vi "magnetoresistance.vi"() -> ()   [LabVIEW 2017]
doc: "Use this template to build a simple state machine design pattern. Each state executes code and determines which state to transition to."
uses:
  controls/State.ctl
  controls/Instruments.ctl
  controls/State_of_loop.ctl
  controls/Data.ctl
  <vilib>/Utility/error.llb/DialogType.ctl
  <vilib>/DAQmx/write.llb/DAQmx Write (Analog DBL 1Chan 1Samp).vi
  <vilib>/DAQmx/create/channels.llb/DAQmx Create Channel (AO-Voltage-Basic).vi
  <vilib>/DAQmx/create/channels.llb/DAQmx Create Channel (AI-Voltage-Basic).vi
  <vilib>/DAQmx/configure/timing.llb/DAQmx Timing (Sample Clock).vi
  <vilib>/DAQmx/configure/trigger.llb/DAQmx Start Trigger (None).vi
  <vilib>/DAQmx/miscellaneous.llb/DAQmx Fill In Error Info.vi
panel:
  in  "Number of loops":i32=1 caption="Stop H Field (Oe)" min=0
  in  "Time to wait, ms":i32=100 caption="Stop H Field (Oe)" min=0
  in  "Clear button":bool
  in  "Data Type":T1(ring)=enum."Resistance, Ohm"
  out "Ush.Min":dbl=-0.5
  out "Ush.Max":dbl=0.5
  out "U.Min":dbl=-0.5
  out "U.Max":dbl=0.5
  in  "Load resistance, Ohm":dbl=2351.0 min=0.0
  in  "Switch port":refnum<visa-resource-name>="COM6"
  in  "AKIP":refnum<visa-resource-name>="AKIP"
  in  "DAQ channel Voltage Output":tag="DAQ6363/ao0"
  in  "DAQ channel Voltage U":tag="DAQ6363/ai5"
  in  "DAQ channel Voltage Ush":tag="DAQ6363/ai4"
  in  "Resolution, Oe/point":dbl=50.0 caption="Stop H Field (Oe)" min=0.0 format="%#_6f"
  out "DC power electromagnet":cluster{"Voltage":dbl, "Current":dbl}={"Voltage"=0.005, "Current"=0.05} {"Voltage" format="%.2f"; "Current" format="%.2f"}
  out "Error Out":errorcluster={"status"=FALSE, "code"=1073676293, "source"="VISA Read in AKIP_read.vi->AKIP_error_check.vi->AKIP_reset_errors.vi->magnetoresistance.vi"}
  in  "Error In (no error)":errorcluster
  in  "Voltage Output, V":dbl=0.5 min=0.0 max=5.0
  in  "H Field Max, Oe":dbl=1200.0 caption="Stop H Field (Oe)" min=0.0 max=6000.0 format="%#_6f"
  in  "H Field Min, Oe":dbl=-1200.0 min=-6000.0 max=0.0 format="%#_6f"
  out "Status":string="Shutting down..."
  in  "Exit Button":bool
  in  "Save Button":bool
  out "Cursor":cluster{"x":dbl, "y":dbl} {"x" format="%.2f"; "y" format="%.5f"}
  out "SpectrumGraph":cluster{"Old Field":dbl[], "Old Signal":dbl[]}[](graph)
  in  "Start Button":bool
  in  "Stop Button":bool
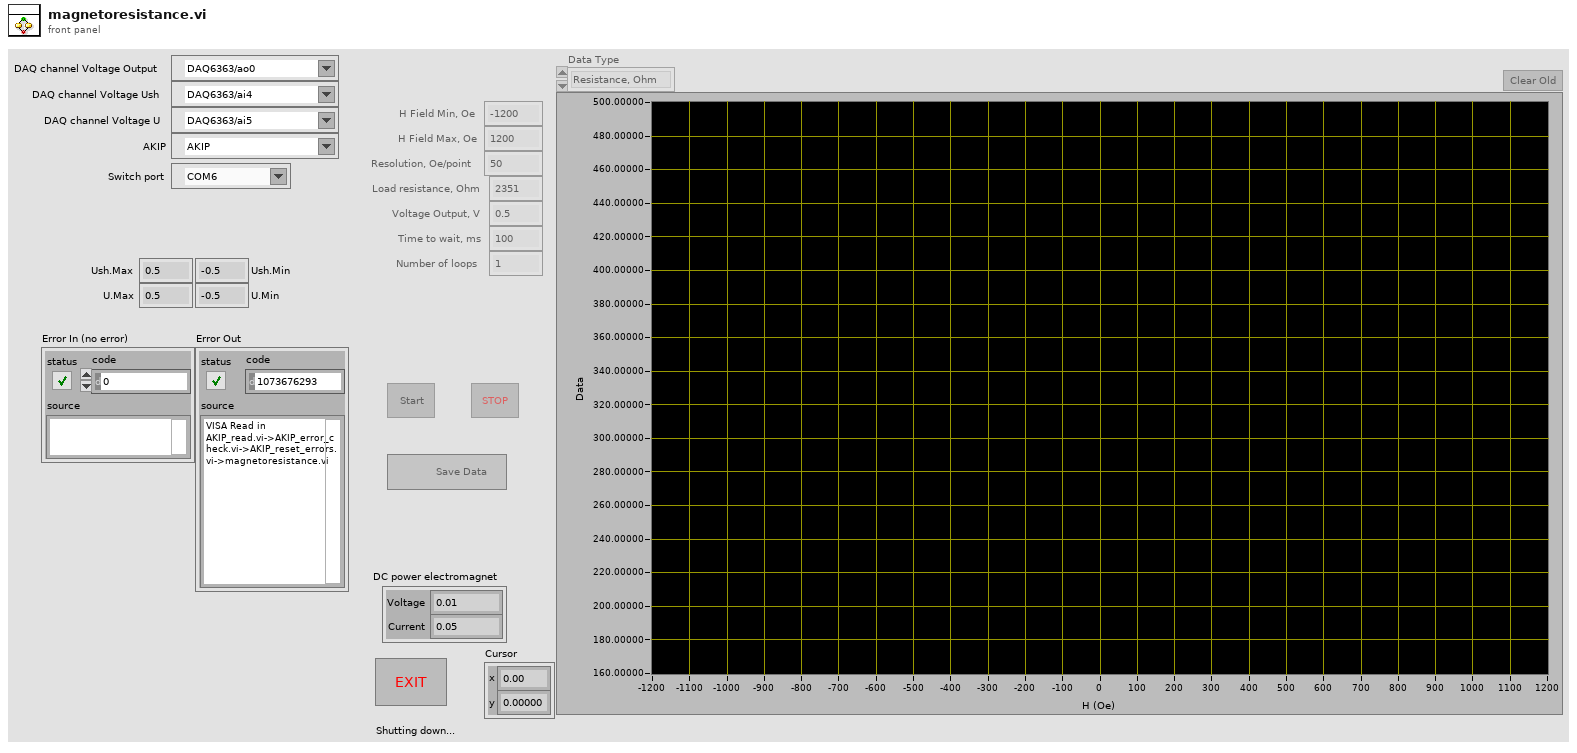
[diagram p1: front panel]
types:
  T1 = enum16{"Voltage Ush, V", "Voltage U, V", "Sum Voltage, V", "Current, mA", "Resistance, Ohm"}
  T2 = typedef "Data.ctl" = cluster{"Field":dbl[], "Voltage Ush":dbl[], "Voltage U":dbl[], "Sum Voltage":dbl[], "Current":dbl[], "Resistance":dbl[], "Old Field":dbl[], "Old Voltage Ush":dbl[], "Old Voltage U":dbl[], "Old Sum Voltage":dbl[], "Old Current":dbl[], "Old Resistance":dbl[]}
  T3 = typedef "State_of_loop.ctl" = enum16{"from zero to max", "from max to zero", "from zero to min", "from min to zero"}
  T4 = typedef "Instruments.ctl" = cluster{"DAQ AO task":refnum<k21>, "DAQ AI task":refnum<k21>, "DAQ channel Voltage Output":tag, "DAQ channel Voltage U":tag, "DAQ channel Voltage Ush":tag, "AKIP":refnum<visa-resource-name>, "Switch port":refnum<visa-resource-name>}
  T5 = typedef "State.ctl" = enum16{"Init", "Idle", "Starting meas", "Running", "Stopping meas", "Shutdown"}
  T6 = cluster{"Old Field":dbl[], "Old Resistance":dbl[]}[]
  T7 = cluster{"Voltage Ush":dbl, "Voltage U":dbl, "Sum Voltage":dbl, "Current":dbl, "Resistance":dbl}
  T8 = typedef "DialogType.ctl" = u16
  T9 = typedef "LVPoint32TypeDef.ctl" = cluster{"Horizontal":i32, "Vertical":i32}
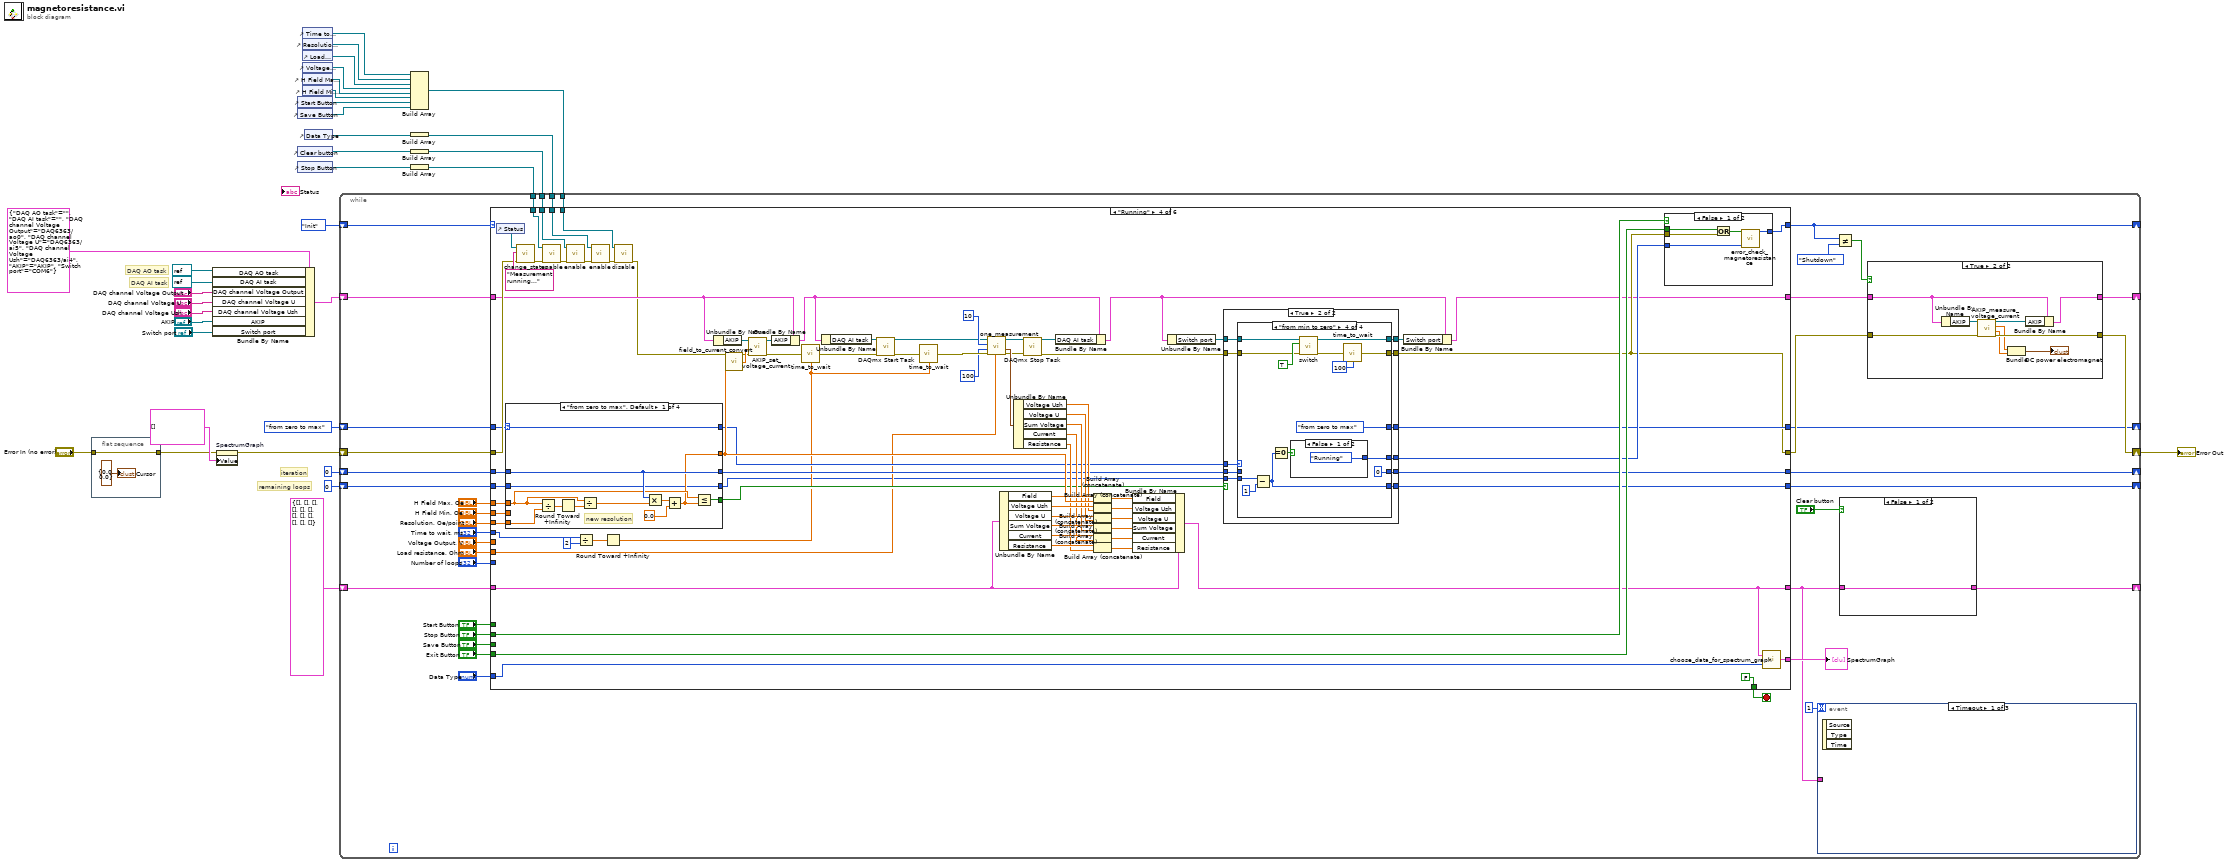
[diagram p0: block diagram]
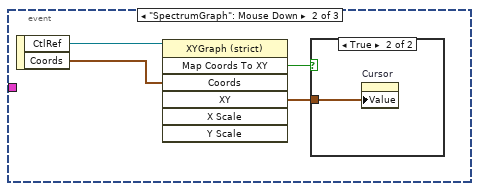
[diagram p3: hidden frame]
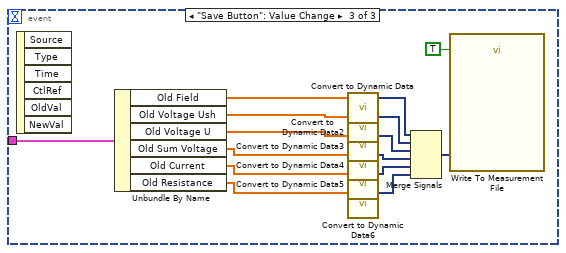
[diagram p5: hidden frame]
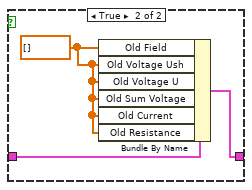
[diagram p6: hidden frame]
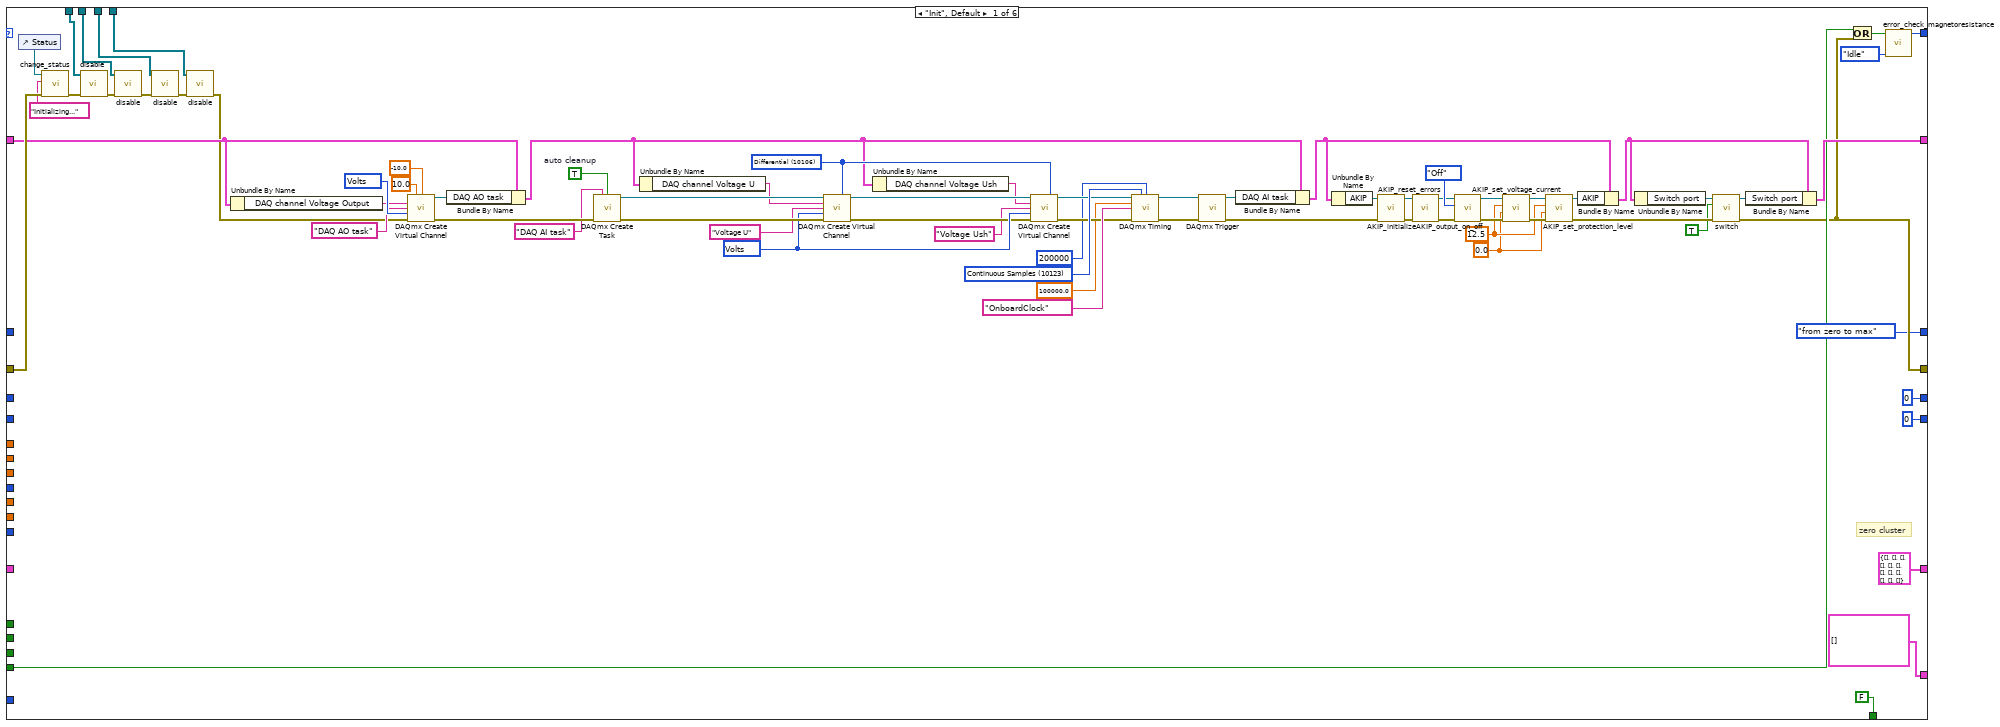
[diagram p7: hidden frame]
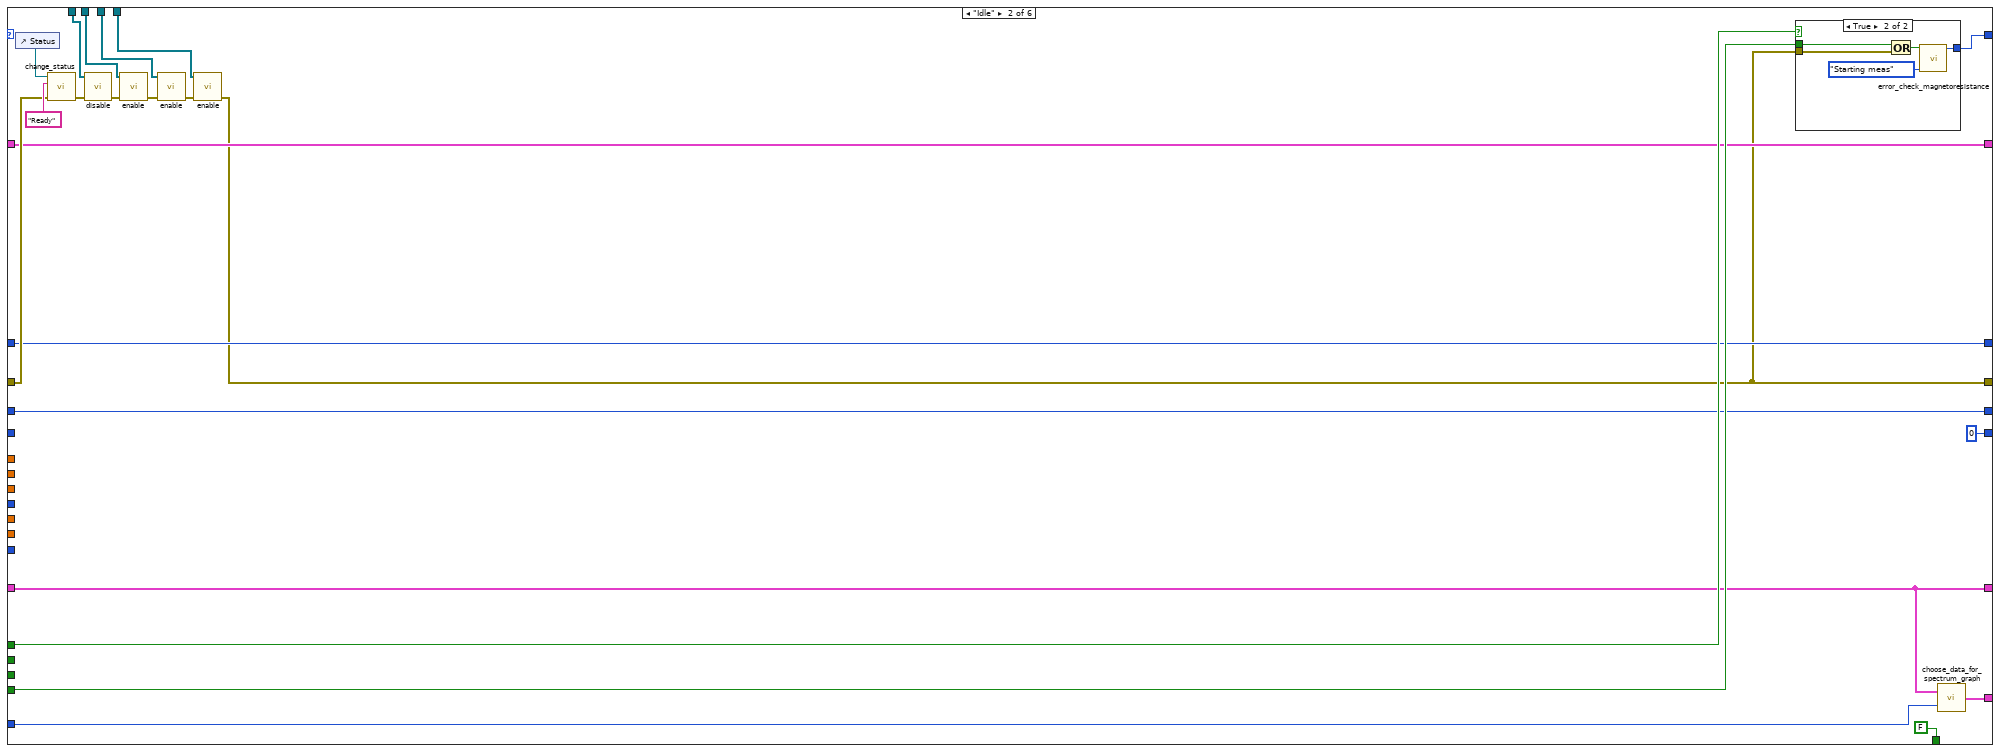
[diagram p8: hidden frame]
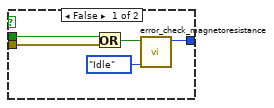
[diagram p9: hidden frame]
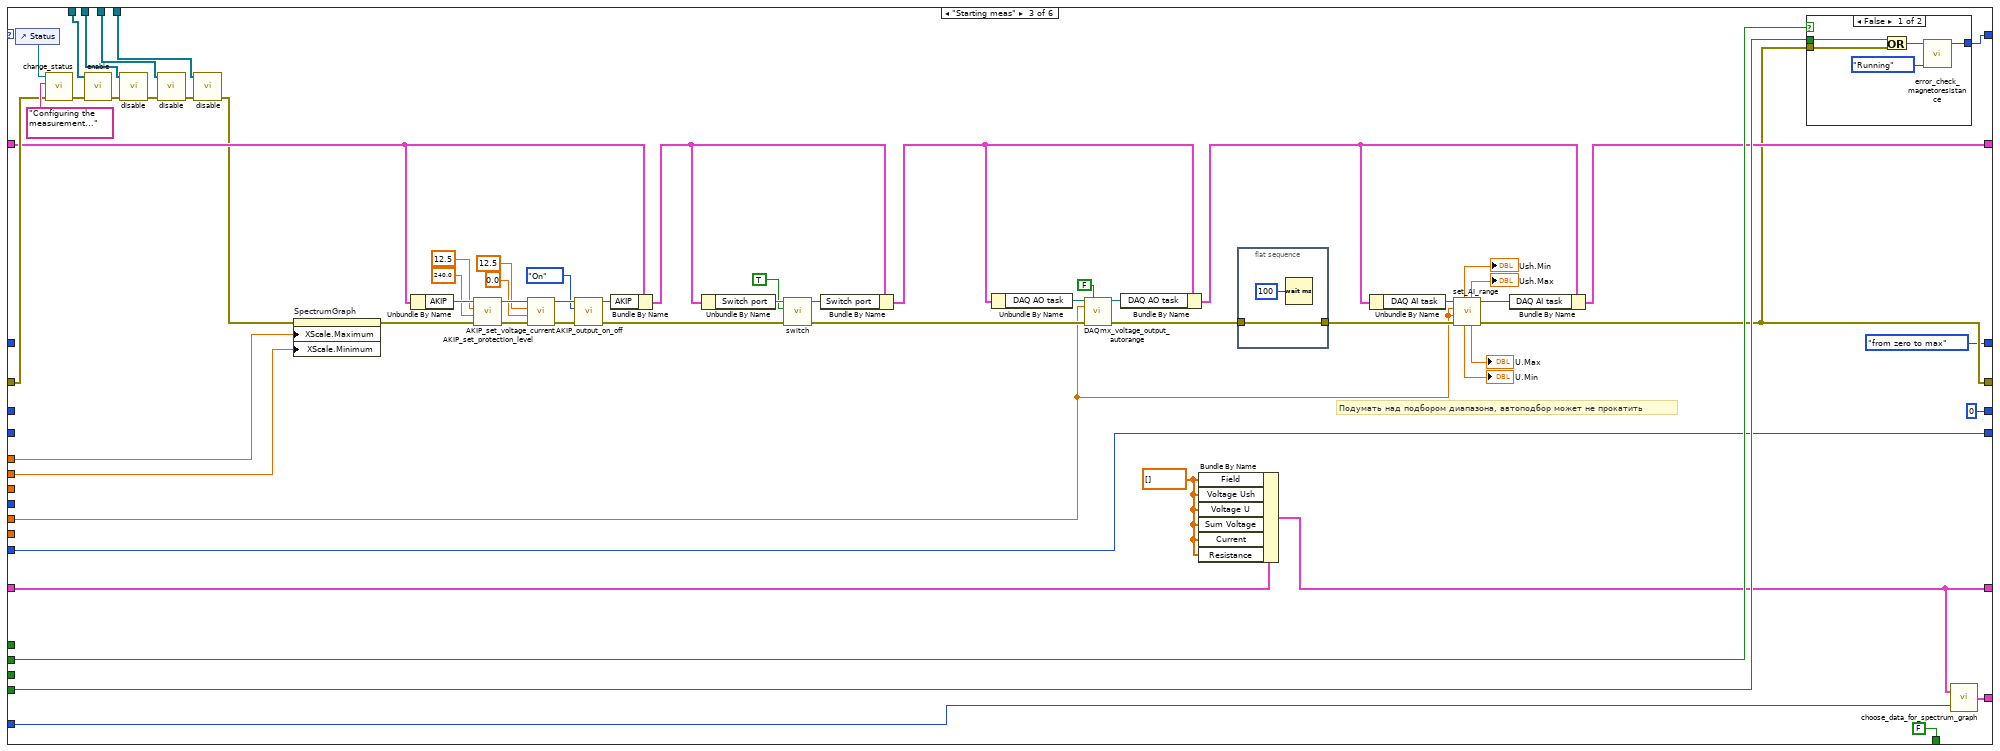
[diagram p10: hidden frame]
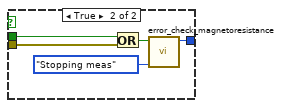
[diagram p11: hidden frame]
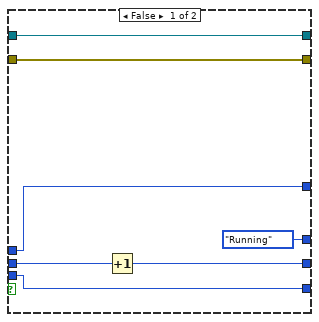
[diagram p12: hidden frame]
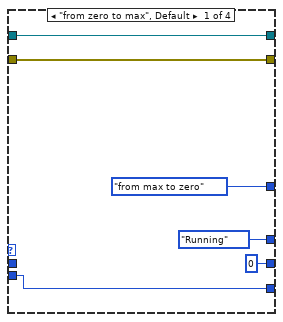
[diagram p13: hidden frame]
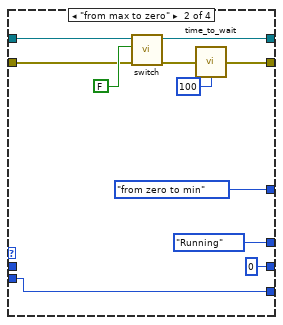
[diagram p14: hidden frame]
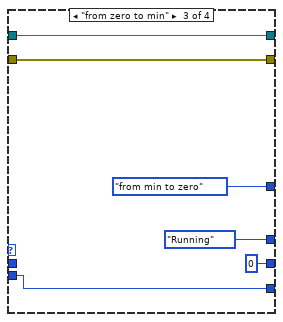
[diagram p15: hidden frame]
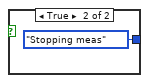
[diagram p16: hidden frame]
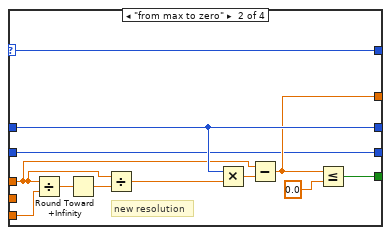
[diagram p17: hidden frame]
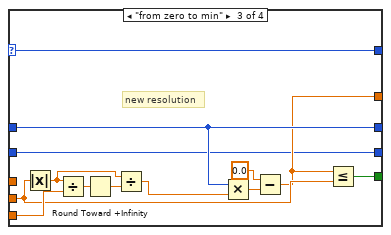
[diagram p18: hidden frame]
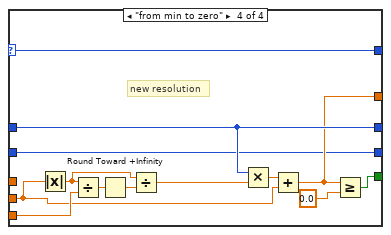
[diagram p19: hidden frame]
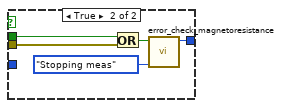
[diagram p20: hidden frame]
diagram:
  # "iteration"
  # "remaining loops"
  # "DAQ AI task"
  # "DAQ AO task"
  n1 = flat-sequence {
    tunnel: "Error In (no error)" -> [w36]
    tunnel: [w36] -> w23
    frame #0 {
      "Cursor" <- cluster{"x":dbl, "y":dbl} {"x"=0.0, "y"=0.0} ("Cursor")
    }
  }
  n2 = Bundle By Name(cluster=T4 {"DAQ AO task"="", "DAQ AI task"="", "DAQ channel Voltage Output"="DAQ6363/ao0", "DAQ channel Voltage U"="DAQ6363/ai5", "DAQ channel Voltage Ush"="DAQ6363/ai4", "AKIP"="AKIP", "Switch port"="COM6"} ("Cluster"), "DAQ AO task"=refnum<k21> refnum ("task in"), "DAQ AI task"=refnum<k21> refnum ("task out"), "DAQ channel Voltage Output"="DAQ channel Voltage Output", "DAQ channel Voltage U"="DAQ channel Voltage U", "DAQ channel Voltage Ush"="DAQ channel Voltage Ush", "AKIP"="AKIP", "Switch port"="Switch port") -> (w15:T4)
  n3 = property on="SpectrumGraph" class="XYGraph (strict)"(error in=w23, "Value"=cluster{"Old Field":dbl[], "Old Signal":dbl[]}[] [] ("SpectrumGraph")) -> (error out=w27:errorcluster)  [unwired: 1 in, 1 out]
  n4 = control-ref of="Start Button"() -> (w32:refnum<vi>)
  n5 = control-ref of="Save Button"() -> (w31:refnum<vi>)
  n6 = control-ref of="Clear button"() -> (w9:refnum<vi>)
  n7 = control-ref of="Stop Button"() -> (w30:refnum<vi>)
  n8 = control-ref of="Time to wait, ms"() -> (w2:refnum<vi>)
  n9 = control-ref of="Resolution, Oe/point"() -> (w3:refnum<vi>)
  n10 = control-ref of="Load resistance, Ohm"() -> (w4:refnum<vi>)
  n11 = control-ref of="Voltage Output, V"() -> (w5:refnum<vi>)
  n12 = control-ref of="H Field Max, Oe"() -> (w34:refnum<vi>)
  n13 = control-ref of="H Field Min, Oe"() -> (w33:refnum<vi>)
  n14 = control-ref of="Data Type"() -> (w8:refnum<vi>)
  n15 = Build Array(w2, w3, w4, w5, w34, w33, w32, w31) -> (w28:refnum<vi>[])
  n16 = Build Array(w8) -> (w7:refnum<vi>[])
  n17 = Build Array(w9) -> (w6:refnum<vi>[])
  n18 = Build Array(w30) -> (w29:refnum<vi>[])
  n19 = while {
    tunnel: w29 -> [w75]
    tunnel: w28 -> [w74]
    shift-right: [w43] -> _
    shift-left: State."Init" ("States") -> [w68]
    shift-right: [w62] -> w14
    shift-left: w27 -> [w73]
    shift-right: [w64] -> _
    shift-left: w15 -> [w66]
    shift-right: [w55] -> _
    shift-left: State_of_loop."from zero to max" -> [w56]
    shift-right: [w53] -> _
    shift-left: 0 -> [w54]
    shift-right: [w48] -> _
    shift-left: T2 {"Field"=[], "Voltage Ush"=[], "Voltage U"=[], "Sum Voltage"=[], "Current"=[], "Resistance"=[], "Old Field"=[], "Old Voltage Ush"=[], "Old Voltage U"=[], "Old Sum Voltage"=[], "Old Current"=[], "Old Resistance"=[]} ("SpectrumGraph") -> [w52]
    tunnel: w6 -> [w45]
    tunnel: w7 -> [w44]
    shift-right: [w37] -> _
    shift-left: 0 -> [w38]
    stop <- w67 stop-if-true
    n20 = case shown="\"Running\"" w68 {
      tunnel: w75 -> [w115 w189 w228 w307 w493 w548]
      tunnel: w74 -> [w112 w186 w225 w304 w490 w545]
      tunnel: w73 -> [w183 w206 w277 w368 w541 w595]
      tunnel: "Start Button" -> [_ w204 _ _ _ _]
      tunnel: "Stop Button" -> [_ _ w252 w366 _ _]
      tunnel: "Save Button" -> [_ _ _ _ _ _]
      tunnel: "Exit Button" -> [w122 w203 w251 w365 w509 _]
      tunnel: [w174 w202 w253 w367 w511 State."Shutdown" ("States out")] -> w43
      tunnel: [FALSE FALSE FALSE FALSE FALSE TRUE] -> w67
      tunnel: w66 -> [w165 w200 w242 w356 w523 w578]
      tunnel: [w123 w200 w249 w319 w514 w570] -> w65
      tunnel: [w121 w190 w248 w323 w510 w577] -> w63
      tunnel: "Load resistance, Ohm" -> [_ _ _ w294 _ _]
      tunnel: "H Field Max, Oe" -> [_ _ w222 w361 _ _]
      tunnel: "H Field Min, Oe" -> [_ _ w221 w360 _ _]
      tunnel: "Voltage Output, V" -> [_ _ w219 _ _ _]
      tunnel: "Resolution, Oe/point" -> [_ _ _ w359 _ _]
      tunnel: w56 -> [_ w199 _ w364 _ _]
      tunnel: [State_of_loop."from zero to max" w199 State_of_loop."from zero to max" w324 State_of_loop."from zero to max" State_of_loop."from zero to max"] -> w55
      tunnel: w54 -> [_ w195 _ w363 _ _]
      tunnel: [0 w195 0 w328 0 0] -> w53
      tunnel: w52 -> [_ w196 w246 w336 w500 _]
      tunnel: [T2 {"Field"=[], "Voltage Ush"=[], "Voltage U"=[], "Sum Voltage"=[], "Current"=[], "Resistance"=[], "Old Field"=[], "Old Voltage Ush"=[], "Old Voltage U"=[], "Old Sum Voltage"=[], "Old Current"=[], "Old Resistance"=[]} ("SpectrumGraph") w196 w244 w316 w499 T2 {"Field"=[], "Voltage Ush"=[], "Voltage U"=[], "Sum Voltage"=[], "Current"=[], "Resistance"=[], "Old Field"=[], "Old Voltage Ush"=[], "Old Voltage U"=[], "Old Sum Voltage"=[], "Old Current"=[], "Old Resistance"=[]} ("SpectrumGraph")] -> w47
      tunnel: [cluster{"Old Field":dbl[], "Old Signal":dbl[]}[] [] w198 w245 w318 w538 T6 [] ("Data for SpectrumGraph")] -> w51
      tunnel: "Data Type" -> [_ w197 w243 w317 w537 _]
      tunnel: w45 -> [w114 w188 w227 w306 w492 w547]
      tunnel: w44 -> [w113 w187 w226 w305 w491 w546]
      tunnel: "Time to wait, ms" -> [_ _ _ w298 _ _]
      tunnel: "Number of loops" -> [_ _ w218 _ _ _]
      tunnel: w38 -> [_ _ _ w293 _ _]
      tunnel: [0 ("Number of loops") 0 ("Number of loops") w218 w291 0 ("Number of loops") 0 ("Number of loops")] -> w37
      frame "Init", Default {
        w130 = 0.0 ("Current")
        w131 = 12.5 ("Voltage")
        w162 = TRUE  # auto cleanup
        w164 = 10123 items=["Finite Samples"=10178, "Continuous Samples"=10123, "Hardware Timed Single Point"=12522] ("sample mode")
        w155 = 10106 items=["Default"=-1, "RSE"=10083, "NRSE"=10078, "Differential"=10106, "Pseudodifferential"=12529] ("input terminal configuration")
        w154 = 10348 items=["Volts"=10348, "From Custom Scale"=10065] ("units")
        w168 = 10348 items=["Volts"=10348, "From Custom Scale"=10065] ("units")
        # "zero cluster"
        n21 = control-ref of="Status"() -> (w184:refnum<vi>)
        n22 = call "change_status.vi"("error in (no error)"=w183, "String"="Initializing...", "String in"=w184) -> ("error out"=w182:errorcluster)  [unwired: 8 in]
        n23 = call "disable.vi"("error in (no error)"=w182, "Array"=w115) -> ("error out"=w181:errorcluster)  [unwired: 9 in]
        n24 = call "disable.vi"("error in (no error)"=w181, "Array"=w114) -> ("error out"=w117:errorcluster)  [unwired: 9 in]
        n25 = call "disable.vi"("error in (no error)"=w117, "Array"=w113) -> ("error out"=w118:errorcluster)  [unwired: 9 in]
        n26 = call "disable.vi"("error in (no error)"=w118, "Array"=w112) -> ("error out"=w116:errorcluster)  [unwired: 9 in]
        n27 = Unbundle By Name(w165) -> ("DAQ channel Voltage Output"=w167:tag)
        n28 = call-poly <vilib>:"DAQmx Create Virtual Channel.vi"("maximum value"=10.0, "minimum value"=-10.0, "physical channels"=w167, "name to assign"="DAQ AO task", "units"=w168, "error in"=w116) -> ("task out"=w166:refnum<k21>, "error out"=w151:errorcluster)  [unwired: 8 in]
        n29 = Bundle By Name(cluster=w165, "DAQ AO task"=w166) -> (w141:T4)
        n30 = call <vilib>:"DAQmx Create Task.vi"("new task name"="DAQ AI task", "auto cleanup"=w162, "error in"=w151) -> ("task out"=w161:refnum<k21>, "error out"=w160:errorcluster)  [unwired: 11 in]
        n31 = Unbundle By Name(w141) -> ("DAQ channel Voltage U"=w147:tag)
        n32 = call-poly <vilib>:"DAQmx Create Virtual Channel.vi"("task in"=w161, "input terminal configuration"=w155, "physical channels"=w147, "name to assign"="Voltage U", "units"=w154, "error in"=w160) -> ("task out"=w153:refnum<k21>, "error out"=w152:errorcluster)  [unwired: 8 in]
        n33 = Unbundle By Name(w141) -> ("DAQ channel Voltage Ush"=w146:tag)
        n34 = call-poly <vilib>:"DAQmx Create Virtual Channel.vi"("task in"=w153, "input terminal configuration"=w155, "physical channels"=w146, "name to assign"="Voltage Ush", "units"=w154, "error in"=w152) -> ("task out"=w159:refnum<k21>, "error out"=w158:errorcluster)  [unwired: 8 in]
        n35 = call-poly <vilib>:"DAQmx Timing.vi"("task/channels in"=w159, "sample mode"=w164, "samples per channel"=200000, "rate"=100000.0, "source"=tag "OnboardClock", "error in"=w158) -> ("task out"=w157:refnum<k21>, "error out"=w156:errorcluster)  [unwired: 8 in]
        n36 = call-poly <vilib>:"DAQmx Trigger.vi"("task/channels in"=w157, "error in"=w156) -> ("task out"=w142:refnum<k21>, "error out"=w139:errorcluster)  [unwired: 12 in]
        n37 = Bundle By Name(cluster=w141, "DAQ AI task"=w142) -> (w138:T4)
        n38 = Unbundle By Name(w138) -> ("AKIP"=w140:refnum<visa-resource-name>)
        n39 = call "AKIP_initialize.vi"("error in (no error)"=w139, "VISA Refnum in"=w140) -> ("error out"=w178:errorcluster, "VISA Refnum out"=w179:refnum<visa-resource-name>)  [unwired: 8 in]
        n40 = call "AKIP_reset_errors.vi"("error in (no error)"=w178, "VISA Refnum in"=w179) -> ("error out"=w177:errorcluster, "VISA Refnum out"=w171:refnum<visa-resource-name>)  [unwired: 8 in]
        n41 = call "AKIP_output_on_off.vi"("error in (no error)"=w177, "Enum"=enum16{"On", "Off"}."Off", "VISA Refnum in"=w171) -> ("error out"=w134:errorcluster, "VISA Refnum out"=w135:refnum<visa-resource-name>)  [unwired: 7 in]
        n42 = call "AKIP_set_voltage_current.vi"("error in (no error)"=w134, "Current"=w130, "Voltage"=w131, "VISA resource name (in)"=w135) -> ("error out"=w133:errorcluster, "VISA resource name (out)"=w132:refnum<visa-resource-name>)  [unwired: 6 in]
        n43 = call "AKIP_set_protection_level.vi"("error in (no error)"=w133, "Current Protection Level"=w130, "Voltage Protection Level"=w131, "VISA resource name (in)"=w132) -> ("error out"=w128:errorcluster, "VISA resource name (out)"=w129:refnum<visa-resource-name>)  [unwired: 6 in]
        n44 = Bundle By Name(cluster=w138, "AKIP"=w129) -> (w124:T4)
        n45 = Unbundle By Name(w124) -> ("Switch port"=w127:refnum<visa-resource-name>)
        n46 = call "switch.vi"("error in (no error)"=w128, "Positive?"=TRUE, "Switch port (in)"=w127) -> ("error out"=w121:errorcluster, "Switch port (out)"=w125:refnum<visa-resource-name>)  [unwired: 7 in]
        n47 = Bundle By Name(cluster=w124, "Switch port"=w125) -> (w123:T4)
        n48 = Or(x=w122, y=w121) -> (x .or. y?=w175:bool)
        n49 = call "error_check_magnetoresistance.vi"("States in"=State."Idle" ("States"), "Boolean"=w175) -> ("States out"=w174:T5)  [unwired: 9 in]
      }
      frame "Idle" {
        n50 = control-ref of="Status"() -> (w205:refnum<vi>)
        n51 = call "change_status.vi"("error in (no error)"=w206, "String"="Ready", "String in"=w205) -> ("error out"=w191:errorcluster)  [unwired: 8 in]
        n52 = call "disable.vi"("error in (no error)"=w191, "Array"=w189) -> ("error out"=w194:errorcluster)  [unwired: 9 in]
        n53 = call "enable.vi"("error in (no error)"=w194, "Array"=w188) -> ("error out"=w192:errorcluster)  [unwired: 9 in]
        n54 = call "enable.vi"("error in (no error)"=w192, "Array"=w187) -> ("error out"=w193:errorcluster)  [unwired: 9 in]
        n55 = call "enable.vi"("error in (no error)"=w193, "Array"=w186) -> ("error out"=w190:errorcluster)  [unwired: 9 in]
        n56 = case shown="True" w204 {
          tunnel: w203 -> [w209 w215]
          tunnel: [w210 w214] -> w202
          tunnel: w190 -> [w208 w213]
          frame False {
            n57 = Or(x=w209, y=w208) -> (x .or. y?=w212:bool)
            n58 = call "error_check_magnetoresistance.vi"("States in"=State."Idle" ("States"), "Boolean"=w212) -> ("States out"=w210:T5)  [unwired: 9 in]
          }
          frame True {
            n59 = Or(x=w215, y=w213) -> (x .or. y?=w217:bool)
            n60 = call "error_check_magnetoresistance.vi"("States in"=State."Starting meas" ("States"), "Boolean"=w217) -> ("States out"=w214:T5)  [unwired: 9 in]
          }
        }
        n61 = call "choose_data_for_spectrum_graph.vi"("Data Type"=w197, "Data cluster"=w196) -> ("Data for SpectrumGraph"=w198:T6)
      }
      frame "Starting meas" {
        w247 = dbl[] [] ("Field")
        # "Подумать над подбором диапазона, автоподбор может не прокатить"
        n62 = control-ref of="Status"() -> (w276:refnum<vi>)
        n63 = call "change_status.vi"("error in (no error)"=w277, "String"="Configuring the measurement...", "String in"=w276) -> ("error out"=w229:errorcluster)  [unwired: 8 in]
        n64 = call "enable.vi"("error in (no error)"=w229, "Array"=w228) -> ("error out"=w232:errorcluster)  [unwired: 9 in]
        n65 = call "disable.vi"("error in (no error)"=w232, "Array"=w227) -> ("error out"=w230:errorcluster)  [unwired: 9 in]
        n66 = call "disable.vi"("error in (no error)"=w230, "Array"=w226) -> ("error out"=w231:errorcluster)  [unwired: 9 in]
        n67 = call "disable.vi"("error in (no error)"=w231, "Array"=w225) -> ("error out"=w223:errorcluster)  [unwired: 9 in]
        n68 = property on="SpectrumGraph" class="XYGraph (strict)"(error in=w223, "XScale.Maximum"=w222, "XScale.Minimum"=w221) -> (error out=w224:errorcluster)  [unwired: 1 in, 1 out]
        n69 = Unbundle By Name(w242) -> ("AKIP"=w271:refnum<visa-resource-name>)
        n70 = call "AKIP_set_protection_level.vi"("error in (no error)"=w224, "Current Protection Level"=240.0 ("Voltage Protection Level"), "Voltage Protection Level"=12.5 ("Current Protection Level"), "VISA resource name (in)"=w271) -> ("error out"=w269:errorcluster, "VISA resource name (out)"=w270:refnum<visa-resource-name>)  [unwired: 6 in]
        n71 = call "AKIP_set_voltage_current.vi"("error in (no error)"=w269, "Current"=0.0, "Voltage"=12.5, "VISA resource name (in)"=w270) -> ("error out"=w262:errorcluster, "VISA resource name (out)"=w263:refnum<visa-resource-name>)  [unwired: 6 in]
        n72 = call "AKIP_output_on_off.vi"("error in (no error)"=w262, "Enum"=enum16{"On", "Off"}."On", "VISA Refnum in"=w263) -> ("error out"=w241:errorcluster, "VISA Refnum out"=w261:refnum<visa-resource-name>)  [unwired: 7 in]
        n73 = Bundle By Name(cluster=w242, "AKIP"=w261) -> (w240:T4)
        n74 = Unbundle By Name(w240) -> ("Switch port"=w266:refnum<visa-resource-name>)
        n75 = call "switch.vi"("error in (no error)"=w241, "Positive?"=TRUE, "Switch port (in)"=w266) -> ("error out"=w220:errorcluster, "Switch port (out)"=w265:refnum<visa-resource-name>)  [unwired: 7 in]
        n76 = Bundle By Name(cluster=w240, "Switch port"=w265) -> (w239:T4)
        n77 = Unbundle By Name(w239) -> ("DAQ AO task"=w273:refnum<k21>)
        n78 = call "DAQmx_voltage_output_autorange.vi"("DAQ task Voltage Output in"=w273, "Bipolar"=FALSE, "Voltage Output, V"=w219, "error in (no error)"=w220) -> ("DAQ task Voltage Output out"=w272:refnum<k21>, "error out"=w236:errorcluster)  [unwired: 8 in, 2 out]
        n79 = Bundle By Name(cluster=w239, "DAQ AO task"=w272) -> (w250:T4)
        n80 = Bundle By Name(cluster=w246, "Field"=w247, "Voltage Ush"=w247, "Voltage U"=w247, "Sum Voltage"=w247, "Current"=w247, "Resistance"=w247) -> (w244:T2)
        n81 = flat-sequence {
          tunnel: w236 -> [w280]
          tunnel: [w280] -> w235
          frame #0 {
            n82 = Wait (ms)(milliseconds to wait=u32 100) -> ()  [unwired: 1 out]
          }
        }
        n83 = Unbundle By Name(w250) -> ("DAQ AI task"=w259:refnum<k21>)
        n84 = call "set_AI_range.vi"("error in (no error)"=w235, "Ush.Max"=w219, "U.Max"=w219, "DAQ task (in)"=w259) -> ("error out"=w248:errorcluster, "DAQ task (out)"=w258:refnum<k21>, "U.Max"=→"U.Max":dbl, "Ush.Max"=→"Ush.Max":dbl, "U.Min"=→"U.Min":dbl, "Ush.Min"=→"Ush.Min":dbl)  [unwired: 2 in]
        n85 = Bundle By Name(cluster=w250, "DAQ AI task"=w258) -> (w249:T4)
        n86 = case shown="False" w252 {
          tunnel: w251 -> [w282 w288]
          tunnel: [w283 w287] -> w253
          tunnel: w248 -> [w281 w286]
          frame False {
            n87 = Or(x=w282, y=w281) -> (x .or. y?=w285:bool)
            n88 = call "error_check_magnetoresistance.vi"("States in"=State."Running" ("States"), "Boolean"=w285) -> ("States out"=w283:T5)  [unwired: 9 in]
          }
          frame True {
            n89 = Or(x=w288, y=w286) -> (x .or. y?=w290:bool)
            n90 = call "error_check_magnetoresistance.vi"("States in"=State."Stopping meas" ("States"), "Boolean"=w290) -> ("States out"=w287:T5)  [unwired: 9 in]
          }
        }
        n91 = call "choose_data_for_spectrum_graph.vi"("Data Type"=w243, "Data cluster"=w244) -> ("Data for SpectrumGraph"=w245:T6)
      }
      frame "Running" {
        n92 = control-ref of="Status"() -> (w369:refnum<vi>)
        n93 = case shown="\"from zero to max\", Default" w364 {
          selector: w364 -> [w429 w441 w453 w466]
          tunnel: w363 -> [w439 w447 w458 w472]
          tunnel: [w439 w447 w458 w472] -> w329
          tunnel: w361 -> [w431 w445 _ _]
          tunnel: w360 -> [_ _ w456 w470]
          tunnel: w359 -> [w434 w448 w460 w473]
          tunnel: [w430 w442 w454 w467] -> w349
          tunnel: [w432 w443 w455 w468] -> w326
          tunnel: [w429 w441 w453 w466] -> w325
          tunnel: w293 -> [w428 w440 w452 w465]
          tunnel: [w428 w440 w452 w465] -> w292
          frame "from zero to max", Default {
            # "new resolution"
            n94 = Divide(x=w431, y=w434) -> (x/y=w435:dbl)
            n95 = Round Toward +Infinity(x=w435) -> (ceil(x): smallest int >= x=w436:dbl)
            n96 = Divide(x=w431, y=w436) -> (x/y=w433:dbl)
            n97 = Multiply(x=w439, y=w433) -> (x*y=w438:dbl)
            n98 = Add(x=w438, y=0.0) -> (x+y=w430:dbl)
            n99 = Less Or Equal?(x=w431, y=w430) -> (x <= y?=w432:bool)
          }
          frame "from max to zero" {
            # "new resolution"
            n100 = Divide(x=w445, y=w448) -> (x/y=w450:dbl)
            n101 = Round Toward +Infinity(x=w450) -> (ceil(x): smallest int >= x=w449:dbl)
            n102 = Divide(x=w445, y=w449) -> (x/y=w451:dbl)
            n103 = Multiply(x=w447, y=w451) -> (x*y=w446:dbl)
            n104 = Subtract(x=w445, y=w446) -> (x-y=w442:dbl)
            n105 = Less Or Equal?(x=w442, y=0.0) -> (x <= y?=w443:bool)
          }
          frame "from zero to min" {
            # "new resolution"
            n106 = Absolute Value(x=w456) -> (abs(x)=w459:dbl)
            n107 = Divide(x=w459, y=w460) -> (x/y=w463:dbl)
            n108 = Round Toward +Infinity(x=w463) -> (ceil(x): smallest int >= x=w462:dbl)
            n109 = Divide(x=w459, y=w462) -> (x/y=w464:dbl)
            n110 = Multiply(x=w458, y=w464) -> (x*y=w461:dbl)
            n111 = Subtract(x=0.0, y=w461) -> (x-y=w454:dbl)
            n112 = Less Or Equal?(x=w454, y=w456) -> (x <= y?=w455:bool)
          }
          frame "from min to zero" {
            # "new resolution"
            n113 = Absolute Value(x=w470) -> (abs(x)=w474:dbl)
            n114 = Divide(x=w474, y=w473) -> (x/y=w476:dbl)
            n115 = Round Toward +Infinity(x=w476) -> (ceil(x): smallest int >= x=w475:dbl)
            n116 = Divide(x=w474, y=w475) -> (x/y=w477:dbl)
            n117 = Multiply(x=w472, y=w477) -> (x*y=w471:dbl)
            n118 = Add(x=w471, y=w470) -> (x+y=w467:dbl)
            n119 = Greater Or Equal?(x=w467, y=0.0) -> (x >= y?=w468:bool)
          }
        }
        n120 = call "change_status.vi"("error in (no error)"=w368, "String"="Measurement running...", "String in"=w369) -> ("error out"=w308:errorcluster)  [unwired: 8 in]
        n121 = call "enable.vi"("error in (no error)"=w308, "Array"=w307) -> ("error out"=w311:errorcluster)  [unwired: 9 in]
        n122 = call "enable.vi"("error in (no error)"=w311, "Array"=w306) -> ("error out"=w309:errorcluster)  [unwired: 9 in]
        n123 = Divide(x=w298, y=2) -> (x/y=w296:dbl)
        n124 = call "enable.vi"("error in (no error)"=w309, "Array"=w305) -> ("error out"=w310:errorcluster)  [unwired: 9 in]
        n125 = Round Toward +Infinity(x=w296) -> (ceil(x): smallest int >= x=w295:dbl)
        n126 = call "disable.vi"("error in (no error)"=w310, "Array"=w304) -> ("error out"=w303:errorcluster)  [unwired: 9 in]
        n127 = Unbundle By Name(w356) -> ("AKIP"=w358:refnum<visa-resource-name>)
        n128 = call "field_to_current_convert.vi"("Field, Oe"=w349) -> ("Current, A"=w350:dbl)
        n129 = call "AKIP_set_voltage_current.vi"("error in (no error)"=w303, "Current"=w350, "VISA resource name (in)"=w358) -> ("error out"=w300:errorcluster, "VISA resource name (out)"=w357:refnum<visa-resource-name>)  [unwired: 7 in]
        n130 = Bundle By Name(cluster=w356, "AKIP"=w357) -> (w353:T4)
        n131 = call "time_to_wait.vi"("error in (no error)"=w300, "milliseconds to wait"=w295) -> ("error out"=w299:errorcluster)
        n132 = Unbundle By Name(w353) -> ("DAQ AI task"=w355:refnum<k21>)
        n133 = call <vilib>:"DAQmx Start Task.vi"("task/channels in"=w355, "error in"=w299) -> ("task out"=w302:refnum<k21>, "error out"=w301:errorcluster)  [unwired: 12 in]
        n134 = call "time_to_wait.vi"("error in (no error)"=w301, "milliseconds to wait"=w295) -> ("error out"=w354:errorcluster)
        n135 = call "one_measurement.vi"("Rsh, Ohm"=w294, "Error (in)"=w354, "Number of points"=100, "time for one scan, ms"=u32 10, "DAQ AI task (in)"=w302) -> ("Error (out)"=w313:errorcluster, "Data"=w342:T7, "DAQ AI task (out)"=w315:refnum<k21>)  [unwired: 4 in]
        n136 = Unbundle By Name(w336) -> ("Field"=w348:dbl[], "Voltage Ush"=w347:dbl[], "Voltage U"=w346:dbl[], "Sum Voltage"=w345:dbl[], "Current"=w344:dbl[], "Resistance"=w343:dbl[])
        n137 = Unbundle By Name(w342) -> ("Voltage Ush"=w341:dbl, "Voltage U"=w340:dbl, "Sum Voltage"=w339:dbl, "Current"=w338:dbl, "Resistance"=w337:dbl)
        n138 = call <vilib>:"DAQmx Stop Task.vi"("task/channels in"=w315, "error in"=w313) -> ("task out"=w314:refnum<k21>, "error out"=w312:errorcluster)  [unwired: 12 in]
        n139 = Bundle By Name(cluster=w353, "DAQ AI task"=w314) -> (w320:T4)
        n140 = Build Array (concatenate)(w348, w349) -> (w335:dbl[])
        n141 = Build Array (concatenate)(w347, w341) -> (w334:dbl[])
        n142 = Build Array (concatenate)(w346, w340) -> (w333:dbl[])
        n143 = Build Array (concatenate)(w345, w339) -> (w332:dbl[])
        n144 = Build Array (concatenate)(w344, w338) -> (w331:dbl[])
        n145 = Build Array (concatenate)(w343, w337) -> (w330:dbl[])
        n146 = Bundle By Name(cluster=w336, "Field"=w335, "Voltage Ush"=w334, "Voltage U"=w333, "Sum Voltage"=w332, "Current"=w331, "Resistance"=w330) -> (w316:T2)
        n147 = Unbundle By Name(w320) -> ("Switch port"=w322:refnum<visa-resource-name>)
        n148 = case shown="True" w326 {
          tunnel: w329 -> [w376 w386]
          tunnel: [w375 w385] -> w328
          tunnel: [State."Running" ("States") w384] -> w327
          tunnel: w325 -> [w374 w388]
          tunnel: [w374 w387] -> w324
          tunnel: w312 -> [w372 w383]
          tunnel: [w372 w382] -> w323
          tunnel: w322 -> [w373 w381]
          tunnel: [w373 w380] -> w321
          tunnel: w292 -> [w371 w379]
          tunnel: [w371 w378] -> w291
          frame False {
            n149 = Increment(x=w376) -> (x+1=w375:i32)
          }
          frame True {
            n150 = case shown="\"from min to zero\"" w388 {
              tunnel: [State_of_loop."from max to zero" State_of_loop."from zero to min" State_of_loop."from min to zero" State_of_loop."from zero to max"] -> w387
              tunnel: w386 -> [_ _ _ _]
              tunnel: [0 0 0 0] -> w385
              tunnel: [State."Running" ("States") State."Running" ("States") State."Running" ("States") w424] -> w384
              tunnel: w383 -> [w392 w401 w409 w422]
              tunnel: [w392 w396 w409 w416] -> w382
              tunnel: w381 -> [w391 w402 w408 w421]
              tunnel: [w391 w400 w408 w420] -> w380
              tunnel: w379 -> [w389 w395 w406 w415]
              tunnel: [w389 w395 w406 w412] -> w378
              frame "from zero to max", Default {
              }
              frame "from max to zero" {
                n151 = call "switch.vi"("error in (no error)"=w401, "Positive?"=FALSE, "Switch port (in)"=w402) -> ("error out"=w397:errorcluster, "Switch port (out)"=w400:refnum<visa-resource-name>)  [unwired: 7 in]
                n152 = call "time_to_wait.vi"("error in (no error)"=w397, "milliseconds to wait"=u32 100) -> ("error out"=w396:errorcluster)
              }
              frame "from zero to min" {
              }
              frame "from min to zero" {
                n153 = Subtract(x=w415, y=1) -> (x-y=w412:i32)
                n154 = Equal To 0?(x=w412) -> (x = 0?=w413:bool)
                n155 = case shown="False" w413 {
                  tunnel: [State."Running" ("States") State."Stopping meas" ("States")] -> w424
                  frame False {
                  }
                  frame True {
                  }
                }
                n156 = call "switch.vi"("error in (no error)"=w422, "Positive?"=TRUE, "Switch port (in)"=w421) -> ("error out"=w417:errorcluster, "Switch port (out)"=w420:refnum<visa-resource-name>)  [unwired: 7 in]
                n157 = call "time_to_wait.vi"("error in (no error)"=w417, "milliseconds to wait"=u32 100) -> ("error out"=w416:errorcluster)
              }
            }
          }
        }
        n158 = Bundle By Name(cluster=w320, "Switch port"=w321) -> (w319:T4)
        n159 = case shown="False" w366 {
          tunnel: w365 -> [w480 w485]
          tunnel: [w481 w484] -> w367
          tunnel: w323 -> [w479 w483]
          tunnel: w327 -> [w478 _]
          frame False {
            n160 = Or(x=w480, y=w479) -> (x .or. y?=w482:bool)
            n161 = call "error_check_magnetoresistance.vi"("States in"=w478, "Boolean"=w482) -> ("States out"=w481:T5)  [unwired: 9 in]
          }
          frame True {
            n162 = Or(x=w485, y=w483) -> (x .or. y?=w487:bool)
            n163 = call "error_check_magnetoresistance.vi"("States in"=State."Stopping meas" ("States"), "Boolean"=w487) -> ("States out"=w484:T5)  [unwired: 9 in]
          }
        }
        n164 = call "choose_data_for_spectrum_graph.vi"("Data Type"=w317, "Data cluster"=w316) -> ("Data for SpectrumGraph"=w318:T6)
      }
      frame "Stopping meas" {
        w498 = dbl[] [] ("Field")
        n165 = control-ref of="Status"() -> (w540:refnum<vi>)
        n166 = call "change_status.vi"("error in (no error)"=w541, "String"="Stopping the measurement...", "String in"=w540) -> ("error out"=w494:errorcluster)  [unwired: 8 in]
        n167 = call "disable.vi"("error in (no error)"=w494, "Array"=w493) -> ("error out"=w497:errorcluster)  [unwired: 9 in]
        n168 = call "disable.vi"("error in (no error)"=w497, "Array"=w492) -> ("error out"=w495:errorcluster)  [unwired: 9 in]
        n169 = call "disable.vi"("error in (no error)"=w495, "Array"=w491) -> ("error out"=w496:errorcluster)  [unwired: 9 in]
        n170 = call "disable.vi"("error in (no error)"=w496, "Array"=w490) -> ("error out"=w489:errorcluster)  [unwired: 9 in]
        n171 = Unbundle By Name(w523) -> ("AKIP"=w536:refnum<visa-resource-name>)
        n172 = call "AKIP_set_voltage_current.vi"("error in (no error)"=w489, "Current"=0.0 ("Voltage Protection Level"), "Voltage"=12.5 ("Current Protection Level"), "VISA resource name (in)"=w536) -> ("error out"=w534:errorcluster, "VISA resource name (out)"=w535:refnum<visa-resource-name>)  [unwired: 6 in]
        n173 = call "AKIP_set_protection_level.vi"("error in (no error)"=w534, "Current Protection Level"=0.0 ("Current"), "Voltage Protection Level"=12.5 ("Voltage"), "VISA resource name (in)"=w535) -> ("error out"=w527:errorcluster, "VISA resource name (out)"=w528:refnum<visa-resource-name>)  [unwired: 6 in]
        n174 = call "AKIP_output_on_off.vi"("error in (no error)"=w527, "Enum"=enum16{"On", "Off"}."Off", "VISA Refnum in"=w528) -> ("error out"=w524:errorcluster, "VISA Refnum out"=w526:refnum<visa-resource-name>)  [unwired: 7 in]
        n175 = Bundle By Name(cluster=w523, "AKIP"=w526) -> (w522:T4)
        n176 = Unbundle By Name(w522) -> ("Switch port"=w531:refnum<visa-resource-name>)
        n177 = call "switch.vi"("error in (no error)"=w524, "Positive?"=TRUE, "Switch port (in)"=w531) -> ("error out"=w518:errorcluster, "Switch port (out)"=w530:refnum<visa-resource-name>)  [unwired: 7 in]
        n178 = Bundle By Name(cluster=w522, "Switch port"=w530) -> (w521:T4)
        n179 = Unbundle By Name(w521) -> ("DAQ AO task"=w517:refnum<k21>)
        n180 = call-poly <vilib>:"DAQmx Write.vi"("task/channels in"=w517, "data"=0.0 ("Voltage Output, V"), "error in"=w518) -> ("task out"=w516:refnum<k21>, "error out"=w510:errorcluster)  [unwired: 10 in, 1 out]
        n181 = Bundle By Name(cluster=w521, "DAQ AO task"=w516) -> (w514:T4)
        n182 = Unbundle By Name(w500) -> ("Field"=w506:dbl[], "Voltage Ush"=w505:dbl[], "Voltage U"=w504:dbl[], "Sum Voltage"=w503:dbl[], "Current"=w502:dbl[], "Resistance"=w501:dbl[])
        n183 = Bundle By Name(cluster=w500, "Field"=w498, "Voltage Ush"=w498, "Voltage U"=w498, "Sum Voltage"=w498, "Current"=w498, "Resistance"=w498, "Old Field"=w506, "Old Voltage Ush"=w505, "Old Voltage U"=w504, "Old Sum Voltage"=w503, "Old Current"=w502, "Old Resistance"=w501) -> (w499:T2)
        n184 = Or(x=w509, y=w510) -> (x .or. y?=w513:bool)
        n185 = call "error_check_magnetoresistance.vi"("States in"=State."Idle" ("States"), "Boolean"=w513) -> ("States out"=w511:T5)  [unwired: 9 in]
        n186 = call "choose_data_for_spectrum_graph.vi"("Data Type"=w537, "Data cluster"=w499) -> ("Data for SpectrumGraph"=w538:T6)
      }
      frame "Shutdown" {
        w560 = 12.5 ("Voltage")
        w559 = 0.0 ("Current")
        w591 = T8 3 items=["no dialog", "OK message", "continue or stop message", "OK message + warnings", "continue/stop + warnings"] ("type of dialog (OK msg:1)")
        # "zero cluster"
        n187 = control-ref of="Status"() -> (w594:refnum<vi>)
        n188 = call "change_status.vi"("error in (no error)"=w595, "String"="Shutting down...", "String in"=w594) -> ("error out"=w549:errorcluster)  [unwired: 8 in]
        n189 = call "disable.vi"("error in (no error)"=w549, "Array"=w548) -> ("error out"=w552:errorcluster)  [unwired: 9 in]
        n190 = call "disable.vi"("error in (no error)"=w552, "Array"=w547) -> ("error out"=w550:errorcluster)  [unwired: 9 in]
        n191 = call "disable.vi"("error in (no error)"=w550, "Array"=w546) -> ("error out"=w551:errorcluster)  [unwired: 9 in]
        n192 = call "disable.vi"("error in (no error)"=w551, "Array"=w545) -> ("error out"=w544:errorcluster)  [unwired: 9 in]
        n193 = Unbundle By Name(w578) -> ("DAQ AI task"=w583:refnum<k21>)
        n194 = call <vilib>:"DAQmx Stop Task.vi"("task/channels in"=w583, "error in"=w544) -> ("task out"=w592:refnum<k21>, "error out"=w593:errorcluster)  [unwired: 12 in]
        n195 = call <vilib>:"DAQmx Clear Task.vi"("task in"=w592, "error in"=w593) -> ("error out"=w584:errorcluster)  [unwired: 13 in]
        n196 = Unbundle By Name(w578) -> ("DAQ AO task"=w582:refnum<k21>)
        n197 = call-poly <vilib>:"DAQmx Write.vi"("task/channels in"=w582, "auto start"=TRUE, "data"=0.0, "error in"=w584) -> ("task out"=w587:refnum<k21>, "error out"=w588:errorcluster)  [unwired: 9 in, 1 out]
        n198 = call <vilib>:"DAQmx Stop Task.vi"("task/channels in"=w587, "error in"=w588) -> ("task out"=w589:refnum<k21>, "error out"=w590:errorcluster)  [unwired: 12 in]
        n199 = call <vilib>:"DAQmx Clear Task.vi"("task in"=w589, "error in"=w590) -> ("error out"=w562:errorcluster)  [unwired: 13 in]
        n200 = Unbundle By Name(w578) -> ("AKIP"=w561:refnum<visa-resource-name>)
        n201 = call "AKIP_set_voltage_current.vi"("error in (no error)"=w562, "Current"=w559, "Voltage"=w560, "VISA resource name (in)"=w561) -> ("error out"=w564:errorcluster, "VISA resource name (out)"=w563:refnum<visa-resource-name>)  [unwired: 6 in]
        n202 = call "AKIP_set_protection_level.vi"("error in (no error)"=w564, "Current Protection Level"=w559, "Voltage Protection Level"=w560, "VISA resource name (in)"=w563) -> ("error out"=w557:errorcluster, "VISA resource name (out)"=w558:refnum<visa-resource-name>)  [unwired: 6 in]
        n203 = call "AKIP_output_on_off.vi"("error in (no error)"=w557, "Enum"=enum16{"On", "Off"}."Off", "VISA Refnum in"=w558) -> ("error out"=w555:errorcluster, "VISA Refnum out"=w556:refnum<visa-resource-name>)  [unwired: 7 in]
        n204 = call "AKIP_reset_errors.vi"("error in (no error)"=w555, "VISA Refnum in"=w556) -> ("error out"=w580:errorcluster, "VISA Refnum out"=w581:refnum<visa-resource-name>)  [unwired: 8 in]
        n205 = call "AKIP_close.vi"("error in (no error)"=w580, "VISA Refnum in"=w581) -> ("error out"=w575:errorcluster, "VISA resource name out"=w579:refnum<visa-resource-name>)  [unwired: 8 in]
        n206 = Bundle By Name(cluster=w578, "AKIP"=w579) -> (w571:T4)
        n207 = Unbundle By Name(w571) -> ("Switch port"=w574:refnum<visa-resource-name>)
        n208 = call "switch.vi"("error in (no error)"=w575, "Positive?"=TRUE, "Switch port (in)"=w574) -> ("error out"=w569:errorcluster, "Switch port (out)"=w572:refnum<visa-resource-name>)  [unwired: 7 in]
        n209 = Bundle By Name(cluster=w571, "Switch port"=w572) -> (w570:T4)
        n210 = call <vilib>:"Simple Error Handler.vi"("type of dialog (OK msg:1)"=w591, "error in (no error)"=w569) -> ("error out"=w577:errorcluster)  [unwired: 3 in, 4 out]
      }
    }
    "SpectrumGraph" <- w51
    n211 = event shown="[0] Timeout" {
      selector: _ -> [_ _ _]
      dyn-events: _ -> [_ _ _]
      timeout: 1 -> [_ _ _]
      tunnel: w47 -> [_ _ w99]
      event Timeout {
        n212 = event-data() -> ()  [unwired: 1 in, 3 out]
      }
      event "SpectrumGraph": Mouse Down {
        n213 = event-data() -> ("CtlRef"=w88:refnum<vi>, "Coords"=w87:T9)  [unwired: 1 in]
        n214 = invoke on="Invoke Node" class="XYGraph (strict)" method="Map Coords To XY"(reference=w88, "Coords"=w87) -> ("Map Coords To XY"=w89:bool, "XY"=w90:cluster{"X":dbl, "Y":dbl})  [unwired: 5 in, 5 out]
        n215 = case shown="True" w89 {
          tunnel: w90 -> [_ w91]
          frame False {
          }
          frame True {
            n216 = property on="Cursor" class="Clust (strict)"("Value"=w91) -> ()  [unwired: 2 in, 2 out]
          }
        }
      }
      event "Save Button": Value Change {
        n217 = event-data() -> ()  [unwired: 1 in, 6 out]
        n218 = Unbundle By Name(w99) -> ("Old Field"=w106:dbl[], "Old Voltage Ush"=w104:dbl[], "Old Voltage U"=w100:dbl[], "Old Sum Voltage"=w98:dbl[], "Old Current"=w97:dbl[], "Old Resistance"=w96:dbl[])
        n219 = call "Convert to Dynamic Data"("Array"=w106) -> ("Dynamic Data Type"=w105:dynamicdata)  [unwired: 3 in]
        n220 = call "Convert to Dynamic Data2"("Array"=w104) -> ("Dynamic Data Type"=w103:dynamicdata)  [unwired: 3 in]
        n221 = call "Convert to Dynamic Data3"("Array"=w100) -> ("Dynamic Data Type"=w101:dynamicdata)  [unwired: 3 in]
        n222 = call "Convert to Dynamic Data4"("Array"=w98) -> ("Dynamic Data Type"=w95:dynamicdata)  [unwired: 3 in]
        n223 = call "Convert to Dynamic Data5"("Array"=w97) -> ("Dynamic Data Type"=w94:dynamicdata)  [unwired: 3 in]
        n224 = call "Convert to Dynamic Data6"("Array"=w96) -> ("Dynamic Data Type"=w93:dynamicdata)  [unwired: 3 in]
        n225 = Merge Signals(w105, w103, w101, w95, w94, w93) -> (w102:dynamicdata)
        n226 = call "Write To Measurement File"("Signals"=w102, "Reset"=TRUE) -> ()  [unwired: 15 in, 3 out]
      }
    }
    n227 = Not Equal?(x=w43, y=State."Shutdown") -> (x != y?=w41:bool)
    n228 = case shown="False" "Clear button" {
      tunnel: w47 -> [w107 w110]
      tunnel: [w107 w109] -> w48
      frame False {
      }
      frame True {
        w108 = dbl[] [] ("Old Field")
        n229 = Bundle By Name(cluster=w110, "Old Field"=w108, "Old Voltage Ush"=w108, "Old Voltage U"=w108, "Old Sum Voltage"=w108, "Old Current"=w108, "Old Resistance"=w108) -> (w109:T2)
      }
    }
    n230 = case shown="True" w41 {
      tunnel: w65 -> [w77 w84]
      tunnel: [w77 w83] -> w64
      tunnel: w63 -> [w76 w82]
      tunnel: [w76 w81] -> w62
      frame False {
      }
      frame True {
        n231 = Unbundle By Name(w84) -> ("AKIP"=w86:refnum<visa-resource-name>)
        n232 = call "AKIP_measure_voltage_current.vi"("error in (no error)"=w82, "VISA Refnum in"=w86) -> ("error out"=w81:errorcluster, "Current"=w79:dbl, "Voltage"=w80:dbl, "VISA Refnum out"=w85:refnum<visa-resource-name>)  [unwired: 6 in]
        n233 = Bundle("Voltage"=w80, "Current"=w79) -> (→"DC power electromagnet":cluster{"Voltage":dbl, "Current":dbl})  [unwired: 1 in]
        n234 = Bundle By Name(cluster=w84, "AKIP"=w85) -> (w83:T4)
      }
    }
  }
  "Error Out" <- w14
